vi "Kick Process.vi"   [LabVIEW 2013]
uses:
  Kick Global.vi
types:
  T1 = cluster{"Move":dbl, "Upper limit switch":bool, "Lower limit switch ":bool, "Fire!":bool}
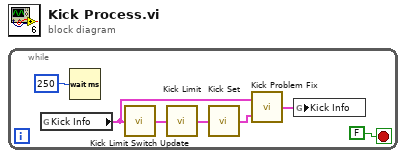
[diagram p0: block diagram]
diagram:
  n1 = while {
    stop <- FALSE stop-if-true
    n2 = global read "Kick Global.vi" "Kick Info"() -> (w2:T1)
    n3 = Wait (ms)(milliseconds to wait=u32 250) -> ()  [unwired: 1 out]
    n4 = call "Kick Limit Switch Update.vi"("Kick Info In"=w2) -> ("Kick Info Out"=w5:T1)
    n5 = call "Kick Limit.vi"("Kick Info In"=w5) -> ("Kick Info Out"=w4:T1)
    n6 = call "Kick Set.vi"("Kick Info In"=w4) -> ("Kick Info Out"=w3:T1)
    n7 = call "Kick Problem Fix.vi"("Kick Info Modified"=w3, "Kick Info Original"=w2) -> ("Kick Info Fixed"=w1:T1)
    n8 = global write "Kick Global.vi" "Kick Info"(w1) -> ()
  }
